vi "stringFirmwareFilter.vi"(8 "error in (no error)":errorcluster, 9 "filter2":string, 10 "inputArray":string[](array[string]), 11 "filter1":string) -> (3 "result string":string)   [LabVIEW 2018]
panel:
  out "error out":errorcluster
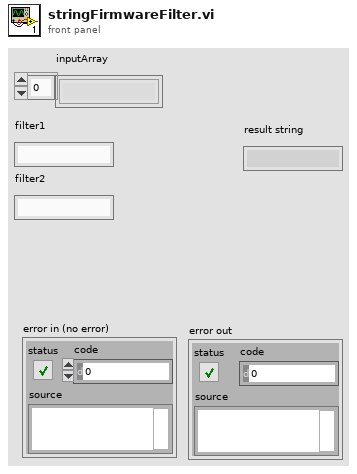
[diagram p1: front panel]
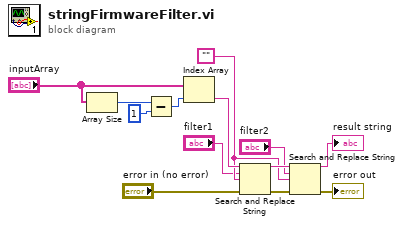
[diagram p0: block diagram]
diagram:
  w8 = ""
  n1 = Array Size(array="inputArray") -> (size(s)=w3:i32)
  n2 = Subtract(x=w3, y=1) -> (x-y=w1:i32)
  n3 = Index Array(array="inputArray", index=w1) -> (element=w13:string)
  n4 = Search and Replace String(input string=w13, search string="filter1", replace string=w8, error in="error in (no error)") -> (result string=w9:string, error out=w10:errorcluster)  [unwired: 4 in, 2 out]
  n5 = Search and Replace String(input string=w9, search string="filter2", replace string=w8, error in=w10) -> (result string=→"result string":string, error out=→"error out":errorcluster)  [unwired: 4 in, 2 out]
